vi "Put Multiple Files and Buffers.vi"(3 "remote port (21)":u16=21, 4 "active (T)":bool=TRUE, 5 "password":string, 7 "user":string="anonymous", 8 "error in (no error)":errorcluster, 9 "timeout ms (60000)":i32=5000, 10 "file specifications":T1(array[cluster]), 11 "host":string) -> (0 "error out":errorcluster, 2 "file errors":errorcluster[](array[cluster]))   [LabVIEW 2023]
uses:
  <vilib>/FTP/NI_FTP.lvlib
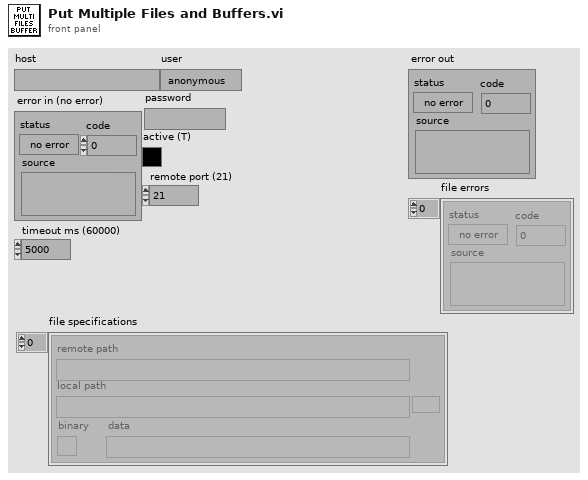
[diagram p1: front panel]
types:
  T1 = cluster{"remote path":string, "local path":path, "binary":bool, "data":string}[]
  T2 = typedef "NI_FTP.lvlib/FTP Session.ctl" = refnum<k5>
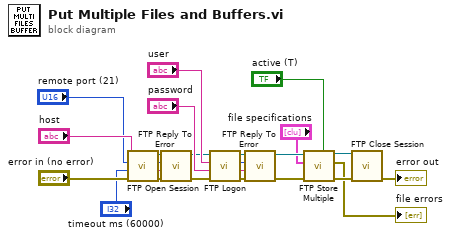
[diagram p0: block diagram]
diagram:
  n1 = call <vilib>:"FTP Open Session.vi"("error in (no error)"="error in (no error)", "timeout ms (60000)"="timeout ms (60000)", "remote port (21)"="remote port (21)", "address"="host") -> ("error out"=w19:errorcluster, "reply string"=w16:string, "reply code"=w17:i32, "ftp session"=w18:T2)  [unwired: 4 out]
  n2 = call <vilib>:"FTP Reply To Error.vi"("error in (no error)"=w19, "reply string in"=w16, "reply code in"=w17, "ftp session"=w18) -> ("error out"=w14:errorcluster, "ftp session out"=w15:T2)  [unwired: 2 out]
  n3 = call <vilib>:"FTP Logon.vi"("error in (no error)"=w14, "password"="password", "user"="user", "ftp session"=w15) -> ("error out"=w13:errorcluster, "reply string"=w10:string, "reply code"=w11:i32, "ftp session out"=w12:T2)  [unwired: 4 out]
  n4 = call <vilib>:"FTP Reply To Error.vi"("error in (no error)"=w13, "reply string in"=w10, "reply code in"=w11, "ftp session"=w12) -> ("error out"=w8:errorcluster, "ftp session out"=w7:T2)  [unwired: 2 out]
  n5 = call <vilib>:"FTP Store Multiple.vi"("active (T)"="active (T)", "error in (no error)"=w8, "file specifications"="file specifications", "ftp session"=w7) -> ("error out"=w9:errorcluster, "file errors"=→"file errors":errorcluster[], "ftp session out"=w5:T2)  [unwired: 5 out]
  n6 = call <vilib>:"FTP Close Session.vi"("error in (no error)"=w9, "ftp session"=w5) -> ("error out"=→"error out":errorcluster)  [unwired: 9 out]
